vi "Set trigger.vi"(8 "error in (no error)":errorcluster, 11 "DAQOrcaFlash in":refnum<class "DAQOrcaFlash.lvclass">) -> (0 "error out":errorcluster, 3 "DAQOrcaFlash out":refnum<class "DAQOrcaFlash.lvclass">)   [LabVIEW 2012, in "DAQOrcaFlash.lvclass"]
uses:
  DAQOrcaFlash.lvclass
  DAQOrcaFlash.lvclass/DAQOrcaFlash.ctl
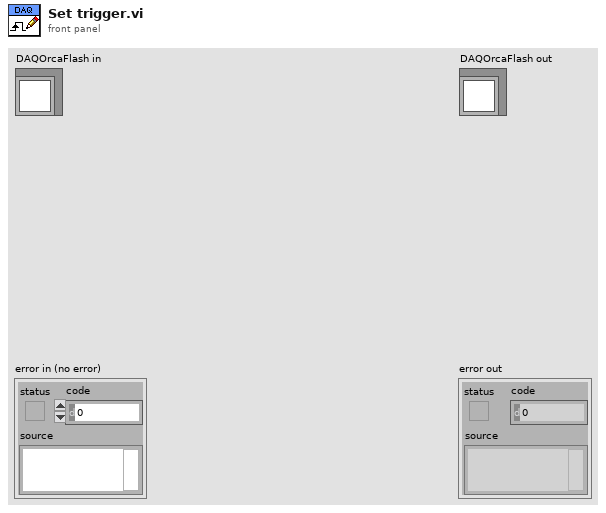
[diagram p1: front panel]
types:
  T1 = typedef "DAQOrcaFlash.lvclass/trigger_mode.ctl" = sgl
  T2 = typedef "DAQOrcaFlash.lvclass/trigger_source.ctl" = sgl
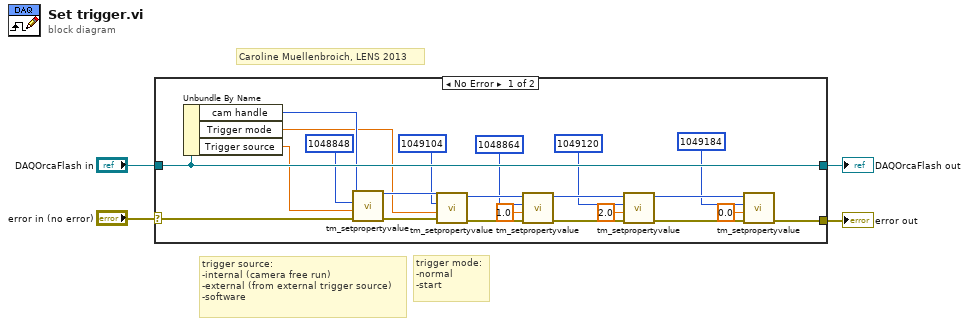
[diagram p0: block diagram]
diagram:
  # "trigger mode:\n-normal\n-start"
  # "trigger source:\n-internal (camera free run) \n-external (from external trigger source)\n-software"
  # "Caroline Muellenbroich, LENS 2013"
  n1 = case shown="No Error" "error in (no error)" {
    selector: "error in (no error)" -> [w21 w28]
    tunnel: [w8 w28] -> w3
    tunnel: [w26 w27] -> w1
    tunnel: "DAQOrcaFlash in" -> [w26 w27]
    frame No Error {
      n2 = Unbundle By Name(w26) -> ("cam handle"=w25:u32, "Trigger mode"=w18:T1, "Trigger source"=w19:T2)
      n3 = call <userlib>:"tm_setpropertyvalue.vi"("error in (no error)"=w21, "Value in"=w19, "Property ID"=u32 1048848, "Handle in"=w25) -> ("error out"=w20:errorcluster, "Handle out"=w24:u32)  [unwired: 6 in]
      n4 = call <userlib>:"tm_setpropertyvalue.vi"("error in (no error)"=w20, "Value in"=w18, "Property ID"=u32 1049104, "Handle in"=w24) -> ("error out"=w17:errorcluster, "Handle out"=w15:u32)  [unwired: 6 in]
      n5 = call <userlib>:"tm_setpropertyvalue.vi"("error in (no error)"=w17, "Value in"=sgl 1.0, "Property ID"=u32 1048864, "Handle in"=w15) -> ("error out"=w16:errorcluster, "Handle out"=w14:u32)  [unwired: 6 in]
      n6 = call <userlib>:"tm_setpropertyvalue.vi"("error in (no error)"=w16, "Value in"=sgl 2.0, "Property ID"=u32 1049120, "Handle in"=w14) -> ("error out"=w9:errorcluster, "Handle out"=w7:u32)  [unwired: 6 in]
      n7 = call <userlib>:"tm_setpropertyvalue.vi"("error in (no error)"=w9, "Value in"=sgl 0.0, "Property ID"=u32 1049184, "Handle in"=w7) -> ("error out"=w8:errorcluster)  [unwired: 6 in, 1 out]
    }
    frame Error {
    }
  }
  "error out" <- w3
  "DAQOrcaFlash out" <- w1
